vi "Remove Sensor.vi"(8 "error in (no error)":errorcluster, 10 "Sensor Enqueuer":refnum<class "Message Enqueuer.lvclass">, 11 "DemoMain in":refnum<class "DemoMain.lvclass">) -> (0 "error out":errorcluster, 3 "DemoMain out":refnum<class "DemoMain.lvclass">)   [LabVIEW 2012, in "Win8uiDemo.lvlib" / "DemoMain.lvclass"]
uses:
  DemoMain.lvclass
  <vilib>/ActorFramework/Message Enqueuer/Message Enqueuer.lvclass
  DemoMain.lvclass/DemoMain.ctl
  <vilib>/ActorFramework/Message Enqueuer/Message Enqueuer.lvclass/Message Enqueuer.ctl
  Read Sensor Enqueuers.vi
  Read GridView Enqueuer.vi
  Write Sensor Enqueuers.vi
  <vilib>/ActorFramework/Message Enqueuer/Enqueue.vi
  <vilib>/ActorFramework/Message Priority Queue/Priority Enqueue.vi
  SubPanel Grid View Messages/Reorder Views Msg/Reorder Views Msg.lvclass
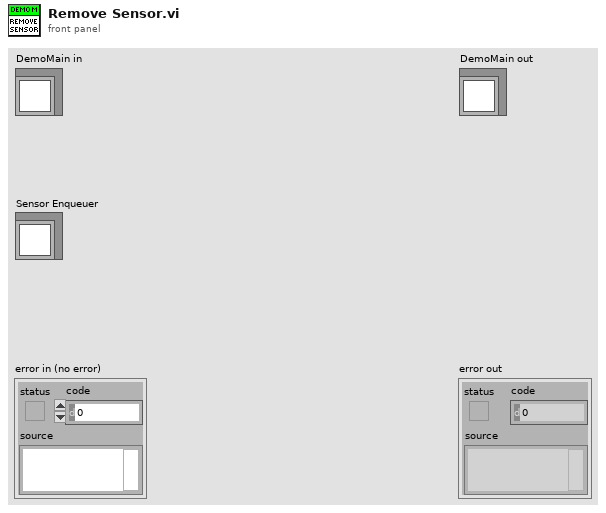
[diagram p1: front panel]
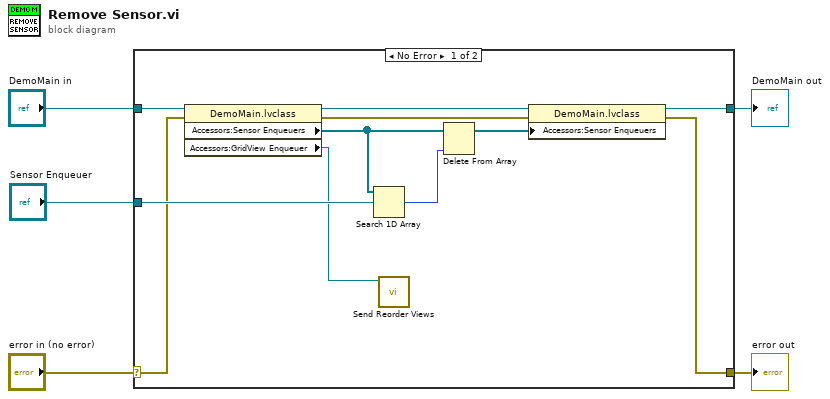
[diagram p0: block diagram]
diagram:
  n1 = case shown="No Error" "error in (no error)" {
    selector: "error in (no error)" -> [w9 w18]
    tunnel: [w7 w18] -> w4
    tunnel: [w15 w17] -> w2
    tunnel: "DemoMain in" -> [w16 w17]
    tunnel: "Sensor Enqueuer" -> [w10 _]
    frame No Error {
      n2 = property class="DemoMain.lvclass"(reference=w16, error in=w9) -> (reference out=w14:refnum<class "DemoMain.lvclass">, error out=w8:errorcluster, "Accessors:Sensor Enqueuers"=w12:refnum<class "Message Enqueuer.lvclass">[], "Accessors:GridView Enqueuer"=w6:refnum<class "Message Enqueuer.lvclass">)
      n3 = Search 1D Array(1D array=w12, element=w10) -> (index of element=w11:i32)  [unwired: 1 in]
      n4 = call "Send Reorder Views.vi"("Message Enqueuer"=w6) -> ()  [unwired: 9 in, 2 out]
      n5 = Delete From Array(array=w12, index=w11) -> (array with subset deleted=w13:refnum<class "Message Enqueuer.lvclass">[])  [unwired: 1 in, 1 out]
      n6 = property class="DemoMain.lvclass"(reference=w14, error in=w8, "Accessors:Sensor Enqueuers"=w13) -> (reference out=w15:refnum<class "DemoMain.lvclass">, error out=w7:errorcluster)
    }
    frame Error {
    }
  }
  "error out" <- w4
  "DemoMain out" <- w2
